vi "Laplace Transform Real.vi"(2 "end":dbl format="%.2f", 3 "X":dbl[](array[numeric])) -> (0 "error":i32, 1 "Laplace {X}":dbl[](array[numeric]))   [LabVIEW 2020, in "NI_Gmath.lvlib"]
doc: "Computes the real Laplace transform of the input sequence <B>X</B>."
uses:
  NI_Gmath.lvlib
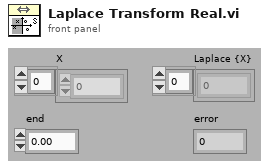
[diagram p1: front panel]
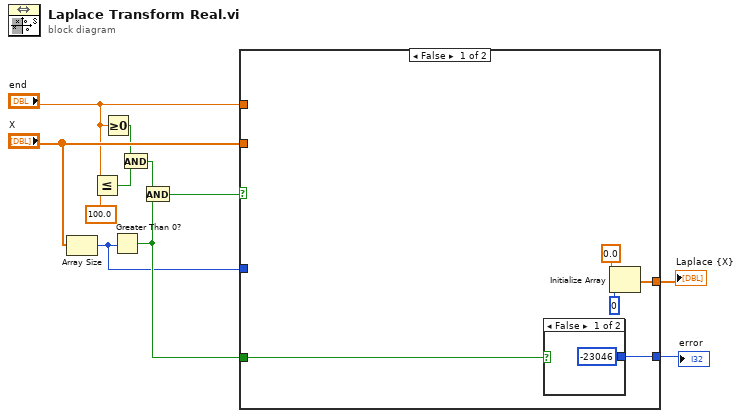
[diagram p0: block diagram]
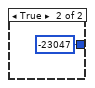
[diagram p2: hidden frame]
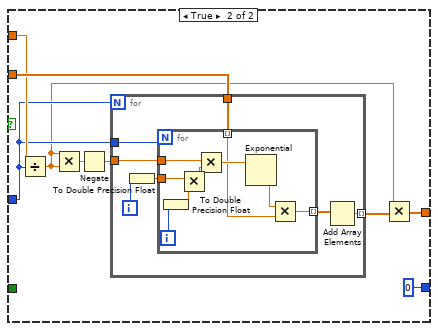
[diagram p3: hidden frame]
diagram:
  n1 = Array Size(array="X") -> (size(s)=w1:i32)
  n2 = Less Or Equal?(x="end", y=100.0) -> (x <= y?=w6:bool)
  n3 = Greater Or Equal To 0?(x="end") -> (x >= 0?=w7:bool)
  n4 = Greater Than 0?(x=w1) -> (x > 0?=w2:bool)
  n5 = And(x=w7, y=w6) -> (x .and. y?=w5:bool)
  n6 = And(x=w5, y=w2) -> (x .and. y?=w4:bool)
  n7 = case shown="False" w4 {
    tunnel: [w14 w19] -> w10
    tunnel: "X" -> [_ w26]
    tunnel: "end" -> [_ w25]
    tunnel: [w12 0] -> w3
    tunnel: w2 -> [w13 _]
    tunnel: w1 -> [_ w22]
    frame False {
      n8 = case shown="False" w13 {
        tunnel: [-23046 -23047] -> w12
        frame False {
        }
        frame True {
        }
      }
      n9 = Initialize Array(0.0, 0) -> (w14:dbl[])
    }
    frame True {
      n10 = Divide(x=w25, y=w22) -> (x/y=w20:dbl)
      n11 = Multiply(x=w20, y=w20) -> (x*y=w24:dbl)
      n12 = Negate(x=w24) -> (-x=w23:dbl)
      n13 = for {
        N: w22 -> [_]
        tunnel: w23 -> [w32]
        tunnel: w26 -> [w31]
        tunnel: [w29] -> w21 mode=indexing
        tunnel: w22 -> [w28]
        i -> [w34]
        n14 = To Double Precision Float(number=w34) -> (double precision float=w33:dbl)
        n15 = for {
          N: w28 -> [_]
          tunnel: w33 -> [w43]
          tunnel: w32 -> [w40]
          tunnel: w31 -> [w36] mode=indexing
          tunnel: [w35] -> w30 mode=indexing
          i -> [w42]
          n16 = To Double Precision Float(number=w42) -> (double precision float=w41:dbl)
          n17 = Multiply(x=w43, y=w41) -> (x*y=w39:dbl)
          n18 = Multiply(x=w40, y=w39) -> (x*y=w38:dbl)
          n19 = Exponential(1:w38) -> (0:w37:dbl)
          n20 = Multiply(x=w37, y=w36) -> (x*y=w35:dbl)
        }
        n21 = Add Array Elements(numeric array=w30) -> (sum=w29:dbl)
      }
      n22 = Multiply(x=w20, y=w21) -> (x*y=w19:dbl[])
    }
  }
  "Laplace {X}" <- w10
  "error" <- w3
